vi "Channel Measurements Add.vi"(7 "WindowNumber":i32 format="%.0g", 8 "error in (no error)":errorcluster {"code" format="%.0x"}, 9 "Name":string, 10 "Channel":string, 11 "instrument handle":refnum<k15>) -> (0 "error out":errorcluster {"code" format="%.0x"}, 2 "Val":i32, 3 "instrument handle out":refnum<k15>)   [LabVIEW 2014, in "Agilent NA.lvlib"]
doc: "Add new measurement in the channel. Return value is the measurement number. Indicated by Tr# on the NA display."
uses:
  Agilent NA.lvlib
  AgNA.dll
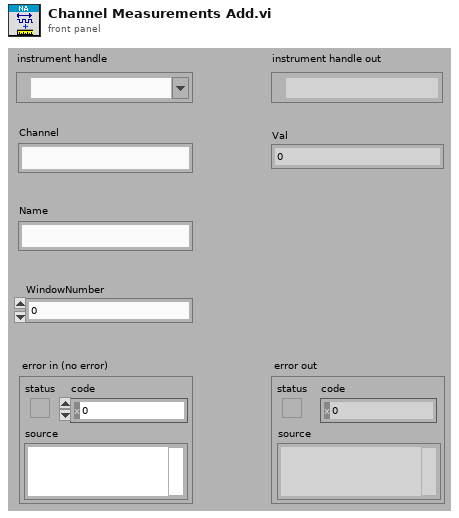
[diagram p1: front panel]
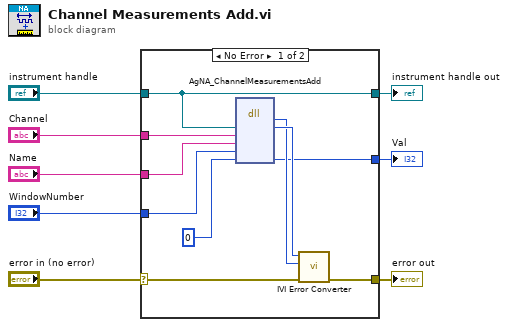
[diagram p0: block diagram]
diagram:
  n1 = case shown="No Error" "error in (no error)" {
    selector: "error in (no error)" -> [w16 w20]
    tunnel: [w15 w20] -> w8
    tunnel: "Channel" -> [w14 _]
    tunnel: "Name" -> [w13 _]
    tunnel: "WindowNumber" -> [w12 _]
    tunnel: [w10 _] -> w3
    tunnel: "instrument handle" -> [w9 w19]
    tunnel: [w9 w19] -> w1
    frame No Error {
      n2 = dll-call lib="AgNA**.dll" fn="AgNA_ChannelMeasurementsAdd"("Vi"=w9, "Channel"=w14, "Name"=w13, "WindowNumber"=w12, "Val"=0) -> (w17:i32, "Vi"=w18:u32, "Val"=w10:i32)  [unwired: 6 in, 2 out]
      n3 = call "IVI Error Converter.vi"("error in (no error)"=w16, "IVI error code (0)"=w17, "instrument handle"=w18) -> ("error out"=w15:errorcluster)  [unwired: 7 in, 1 out]
    }
    frame Error {
    }
  }
  "error out" <- w8
  "instrument handle out" <- w1
  "Val" <- w3
